vi "select_initial_historian.vi"(8 "time_max":timestamp, 9 "time_min":timestamp, 10 "Column table":string[](array[string]), 11 "table":string) -> (3 "parameters":string)   [LabVIEW 2019, in "PostgreSQL.lvlib"]
uses:
  PostgreSQL.lvlib
panel:
  out "Data to write":bool
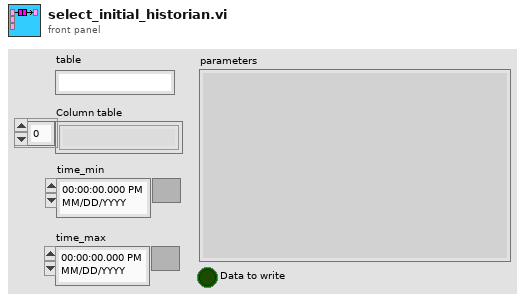
[diagram p1: front panel]
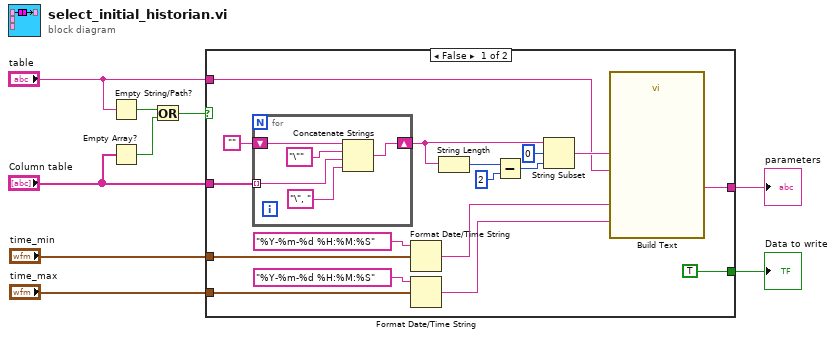
[diagram p0: block diagram]
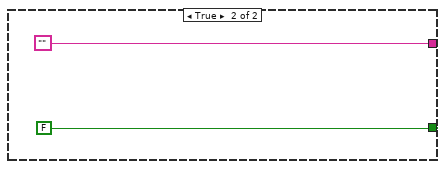
[diagram p2: hidden frame]
diagram:
  n1 = Empty String/Path?(string/path="table") -> (empty?=w6:bool)
  n2 = Empty Array?(array="Column table") -> (empty?=w5:bool)
  n3 = Or(x=w6, y=w5) -> (x .or. y?=w4:bool)
  n4 = case shown="False" w4 {
    tunnel: [w16 ""] -> w9
    tunnel: "table" -> [w17 _]
    tunnel: "Column table" -> [w20 _]
    tunnel: [TRUE FALSE] -> w3
    tunnel: "time_min" -> [w13 _]
    tunnel: "time_max" -> [w11 _]
    frame False {
      n5 = for {
        shift-right: [w29] -> w26
        shift-left: "" -> [w27]
        tunnel: w20 -> [w28] mode=indexing
        n6 = Concatenate Strings(w27, "\"" ("table"), w28, "\", " ("table")) -> (w29:string)
      }
      n7 = Format Date/Time String(time format string (%c)="%Y-%m-%d %H:%M:%S", seconds (now)=w13) -> (date/time string=w14:string)  [unwired: 1 in]
      n8 = Format Date/Time String(time format string (%c)="%Y-%m-%d %H:%M:%S", seconds (now)=w11) -> (date/time string=w10:string)  [unwired: 1 in]
      n9 = String Length(string=w26) -> (length=w25:i32)
      n10 = Subtract(x=w25, y=2) -> (x-y=w23:i32)
      n11 = String Subset(string=w26, offset (0)=0, length (rest)=w23) -> (substring=w18:string)
      n12 = call "Build Text"("time_max"=w10, "columns"=w18, "table"=w17, "time_min"=w14) -> ("Result"=w16:string)  [unwired: 10 in, 1 out]
    }
    frame True {
    }
  }
  "parameters" <- w9
  "Data to write" <- w3
